vi "DualCore.vi"(0 "ref_alphaA":sgl, 1 "ref_max":sgl=0.9999695, 2 "Parameters":T2={"Deadtime"="Deadtime", "Period"="Period"}, 5 "ref_betaA":sgl, 7 "ref_alphaB":sgl, 9 "ref_betaB":sgl, 11 "input valid":bool=TRUE, 12 "enableA":bool=TRUE, 13 "enableB":bool=TRUE) -> (4 "SwitchPositionsA":T1, 6 "SwitchPositionsB":T1, 14 "ready for input":bool, 15 "output valid":bool)   [LabVIEW 2017, in "SVPWM.lvlib"]
uses:
  SVPWM.lvlib
  Parameters.ctl
  SwitchPositions.ctl
  <vilib>/rvi/DataTransferAndStorage/Container/Common/niFpgaContainerExecOnDevCompGetState.vi
  <vilib>/rvi/Emulation/niFpgaEmulationIsFPGAContextNoSignature.vi
  <vilib>/rvi/DataTransferAndStorage/Container/Common/niFpgaContainerGetUniqueNameForEmu.vi
  <vilib>/rvi/Memory/Memory_Emulation/niFpgaMemoryEmulationCacheClearOnFirstRun.vi
  <vilib>/rvi/Memory/Memory_Emulation/nirvimemoryEmulationManagerCache_MakeExclusive.vi
  <vilib>/rvi/Memory/Memory_Emulation/niFpgaMemoryEmulationValidateCache.vi
  <vilib>/rvi/Memory/Memory_Emulation/nirvimemoryEmulationManagerCache_InsertValue.vi
  <vilib>/Utility/error.llb/Clear Errors.vi
  <vilib>/rvi/Memory/Memory_Emulation/nirvimemoryEmulationManagerCache_ReleaseExclusive.vi
  <vilib>/rvi/Memory/Memory_Emulation/nirvimemoryEmulationManagerCache_GetValue.vi
  <vilib>/rvi/Memory/Memory_Emulation/nirvimemoryEmulationManagerCache_SetValue.vi
  <vilib>/rvi/Emulation/niFpgaProcessEmulError.vi
  <vilib>/rvi/Emulation/niFpgaSctlEmulationGetInTimedLoop.vi
  <vilib>/rvi/DataTransferAndStorage/Container/XNode/niFpgaContainer.xnode
  <vilib>/rvi/DataTransferAndStorage/Register/Emulation/niFpgaRegisterEmulationRefIn.vi
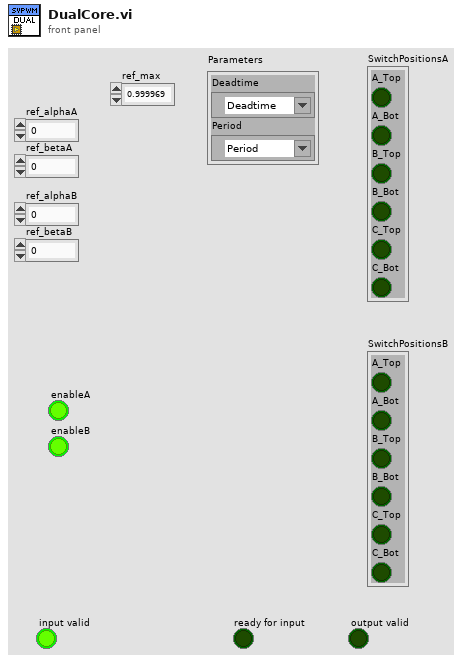
[diagram p1: front panel]
types:
  T1 = typedef "SVPWM.lvlib/SwitchPositions.ctl" = cluster{"A_Top":bool, "A_Bot":bool, "B_Top":bool, "B_Bot":bool, "C_Top":bool, "C_Bot":bool}
  T2 = typedef "SVPWM.lvlib/Parameters.ctl" = cluster{"Deadtime":refnum<k21>, "Period":refnum<k21>}
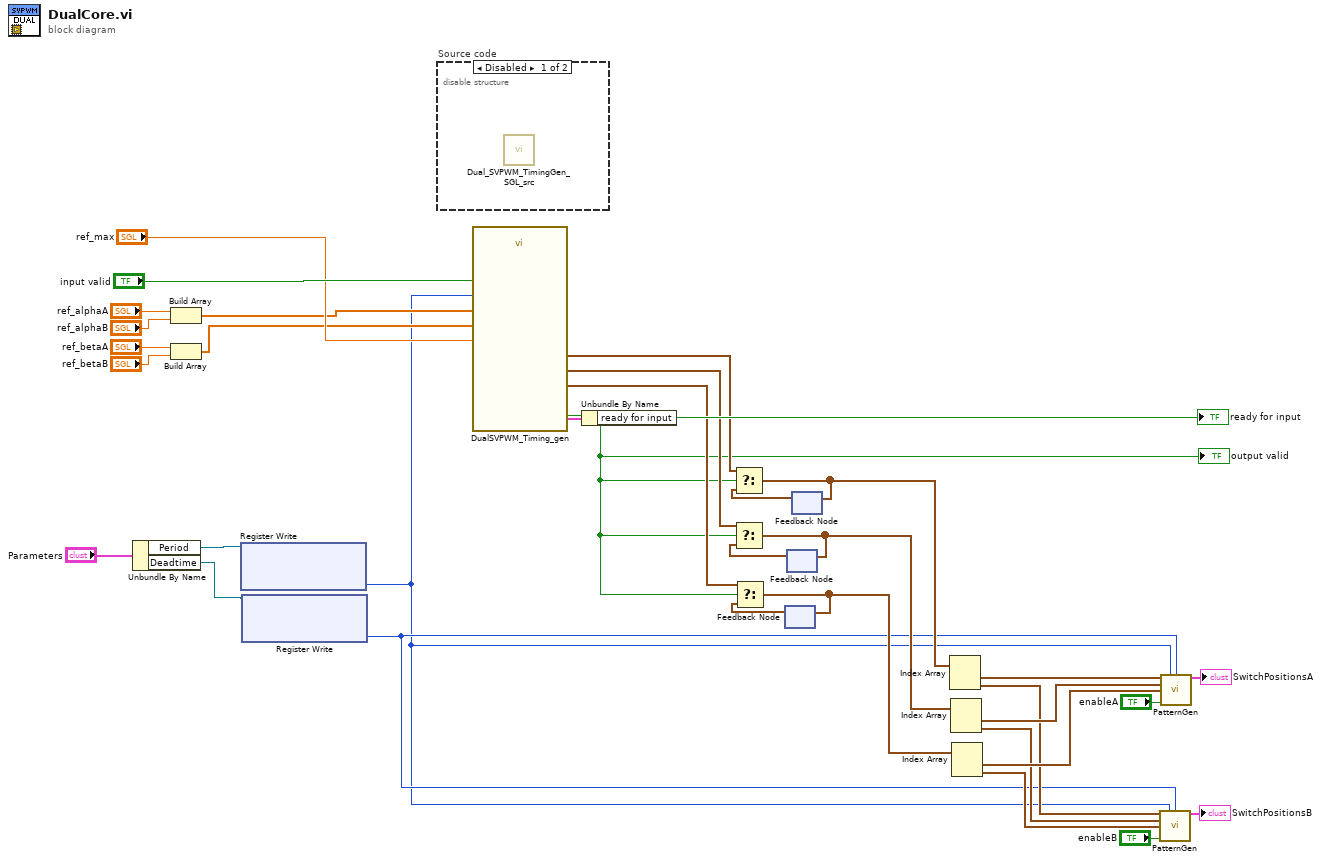
[diagram p0: block diagram]
diagram:
  n1 = Unbundle By Name("Parameters") -> ("Period"=w2:refnum<k21>, "Deadtime"=w4:refnum<k21>)
  n2 = Build Array("ref_alphaA", "ref_alphaB") -> (w20:sgl[])
  n3 = Build Array("ref_betaA", "ref_betaB") -> (w17:sgl[])
  n4 = xnode "Register Write"("Register In"=w2) -> ("Data"=w1:u32)  [unwired: 1 out]
  n5 = xnode "Register Write"("Register In"=w4) -> ("Data"=w3:u8)  [unwired: 1 out]
  n6 = disable-structure "Source code" shown="Disabled" {
    frame Disabled {
      n7 = call "Dual_SVPWM_TimingGen_SGL_src.vi"() -> ()  [unwired: 13 in, 3 out]
    }
    frame Enabled {
    }
  }
  n8 = call "DualSVPWM_Timing_gen.vi"("ref_beta"=w17, "Period"=w1, "ref_max"="ref_max", "input valid"="input valid", "ref_alpha"=w20) -> ("C_timing"=w12:cluster{"ON":u32, "OFF":u32}[], "B_timing"=w13:cluster{"ON":u32, "OFF":u32}[], "A_timing"=w14:cluster{"ON":u32, "OFF":u32}[], "output valid"=w11:bool, "feedback signals"=w16:cluster{"ready for input":bool})  [unwired: 6 in]
  "output valid" <- w11
  n9 = Unbundle By Name(w16) -> ("ready for input"=→"ready for input":bool)
  n10 = feedback #1() -> (w9:cluster{"ON":u32, "OFF":u32}[])  [unwired: 1 in]
  n11 = Select(t=w12, s=w11, f=w9) -> (s? t:f=w5:cluster{"ON":u32, "OFF":u32}[])
  n12 = feedback-in #1(w5) -> ()
  n13 = feedback #2() -> (w8:cluster{"ON":u32, "OFF":u32}[])  [unwired: 1 in]
  n14 = Select(t=w13, s=w11, f=w8) -> (s? t:f=w6:cluster{"ON":u32, "OFF":u32}[])
  n15 = feedback-in #2(w6) -> ()
  n16 = feedback #3() -> (w10:cluster{"ON":u32, "OFF":u32}[])  [unwired: 1 in]
  n17 = Select(t=w14, s=w11, f=w10) -> (s? t:f=w7:cluster{"ON":u32, "OFF":u32}[])
  n18 = feedback-in #3(w7) -> ()
  n19 = Index Array(array=w7) -> (element #1=w32:cluster{"ON":u32, "OFF":u32}, element #2=w29:cluster{"ON":u32, "OFF":u32})  [unwired: 2 in]
  n20 = Index Array(array=w6) -> (element #1=w31:cluster{"ON":u32, "OFF":u32}, element #2=w28:cluster{"ON":u32, "OFF":u32})  [unwired: 2 in]
  n21 = Index Array(array=w5) -> (element #1=w30:cluster{"ON":u32, "OFF":u32}, element #2=w27:cluster{"ON":u32, "OFF":u32})  [unwired: 2 in]
  n22 = call "PatternGen.vi"("A_timing"=w29, "Period"=w1, "Deadtime"=w3, "B_timing"=w28, "C_timing"=w27, "enable"="enableB") -> ("SwitchPositions"=→"SwitchPositionsB":T1)  [unwired: 9 in]
  n23 = call "PatternGen.vi"("A_timing"=w32, "Period"=w1, "Deadtime"=w3, "B_timing"=w31, "C_timing"=w30, "enable"="enableA") -> ("SwitchPositions"=→"SwitchPositionsA":T1)  [unwired: 9 in]
